vi "AddMultipleOperations.vi"(6 "Timeout in ms (-1)":i32, 7 "At opposite end? (F)":bool, 8 "error in (no error)":errorcluster, 10 "Operations":T1[](array[typedef]), 11 "SMP in":refnum<class "SMP.lvclass">) -> (0 "error out":errorcluster, 3 "SMP out":refnum<class "SMP.lvclass">)   [LabVIEW 2013, in "SMP.lvclass"]
doc: "Adds multiple individual operations, to the internal operations queue of the SMP object. These operations are NOT grouped together into a pipe.\n\n<b>At opposite end?: </b>Set to TRUE to add the operations to the front of the internal operations queue. Default is FALSE. The operations are automatically inserted in an inverse order at the front of the queue, such that they will be retrieved in the same order as that in which they are provided to this function.\n\n<b>Operations: </b>The operations to be added. Each operation has a name and data associated with it. Use this Data field to provide any data that the operation needs, except data produced by the operation which executes before it.\n\n<b>Timeout: </b>A timeout for the enqueue operation. Default is -1 (never time out)."
uses:
  SMP.lvclass
  Data types/operation.ctl
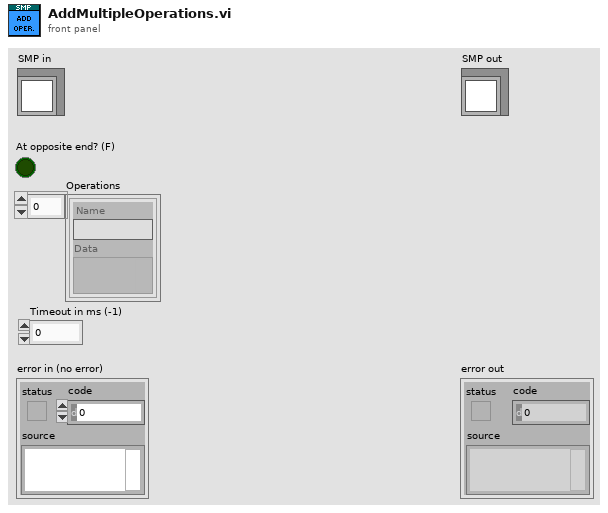
[diagram p1: front panel]
types:
  T1 = typedef "SMP.lvclass/operation.ctl" = cluster{"Name":string, "Data":variant}
  T2 = typedef "Pipe and Filter.lvclass/classData.ctl" = cluster{"Q ref":refnum<queue>, "Previous data":variant, "Current pipe":T3[]}
  T3 = typedef "Pipe and Filter.lvclass/operation.ctl" = cluster{"Name":string, "Data":variant}
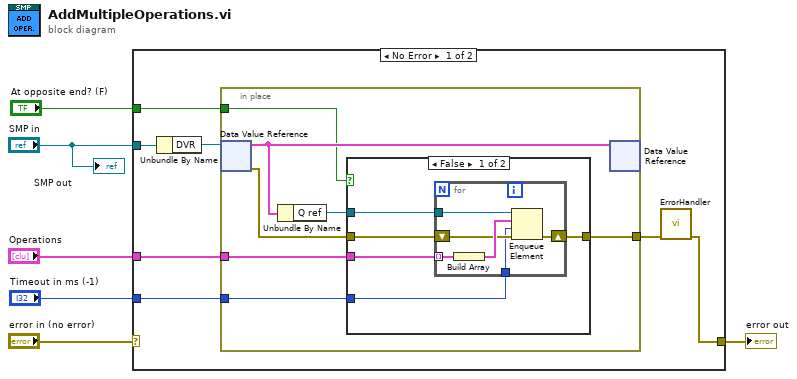
[diagram p0: block diagram]
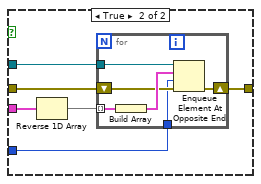
[diagram p2: hidden frame]
diagram:
  n1 = case shown="No Error" "error in (no error)" {
    selector: "error in (no error)" -> [_ w44]
    tunnel: [w9 w44] -> w5
    tunnel: "SMP in" -> [w12 _]
    tunnel: "Operations" -> [w11 _]
    tunnel: "At opposite end? (F)" -> [w8 _]
    tunnel: "Timeout in ms (-1)" -> [w7 _]
    frame No Error {
      n2 = Unbundle By Name(w12) -> ("DVR"=w13:refnum<data-value>)
      n3 = in-place {
        in-place-border: w11 -> [w18]
        in-place-border: [w17] -> w10
        in-place-border: w8 -> [w15]
        in-place-border: w7 -> [w14]
        n4 = in-place-dvr #1(w13) -> (w20:T2, w16:errorcluster)
        n5 = Unbundle By Name(w20) -> ("Q ref"=w19:refnum<queue>)
        n6 = case shown="False" w15 {
          tunnel: w19 -> [w25 w37]
          tunnel: w18 -> [w24 w36]
          tunnel: [w23 w35] -> w17
          tunnel: w16 -> [w22 w34]
          tunnel: w14 -> [w21 w32]
          frame False {
            n7 = for {
              tunnel: w25 -> [w31]
              tunnel: w24 -> [w30] mode=indexing
              shift-right: [w28] -> w23
              shift-left: w22 -> [w27]
              tunnel: w21 -> [w26]
              n8 = Build Array(w30) -> (w29:T1[])
              n9 = Enqueue Element(queue=w31, element=w29, timeout in ms (-1)=w26, error in (no error)=w27) -> (error out=w28:errorcluster)  [unwired: 2 out]
            }
          }
          frame True {
            n10 = Reverse 1D Array(array=w36) -> (reversed array=w33:T1[])
            n11 = for {
              tunnel: w37 -> [w43]
              tunnel: w33 -> [w42] mode=indexing
              shift-right: [w40] -> w35
              shift-left: w34 -> [w39]
              tunnel: w32 -> [w38]
              n12 = Build Array(w42) -> (w41:T1[])
              n13 = Enqueue Element At Opposite End(queue=w43, element=w41, timeout in ms (-1)=w38, error in (no error)=w39) -> (error out=w40:errorcluster)  [unwired: 2 out]
            }
          }
        }
        n14 = in-place-dvr #1(w20) -> ()  [unwired: 2 out]
      }
      n15 = call "ErrorHandler.vi"("error in (no error)"=w10) -> ("error out"=w9:errorcluster)  [unwired: 9 in, 1 out]
    }
    frame Error {
    }
  }
  "error out" <- w5
  "SMP out" <- "SMP in"
